vi "Calculate Zoom from ROI & Image Size.vi"(8 "Error In":errorcluster, 10 "ROI Descriptor":T1 {"Contours"."Type" items=["No Selection", "Point", "Line", "Rectangle", "Oval", "Polygon", "Freehand Region", "Annulus", "Unused2", "Unused3", "Broken Line", "Freehand Line", "Rotated Rectangle"]}, 11 "Displayed Image:Size":cluster{"Width":u32, "Height":u32}) -> (0 "Error Out":errorcluster, 2 "Center Position":cluster{dbl, dbl}, 3 "Zoom Factor":cluster{dbl, dbl})   [LabVIEW 2021, in "Image.lvlib"]
uses:
  <vilib>/Utility/error.llb/Error Cluster From Error Code.vi
  <vilib>/ErrorRing/Error Ring.xnode
  Image.lvlib
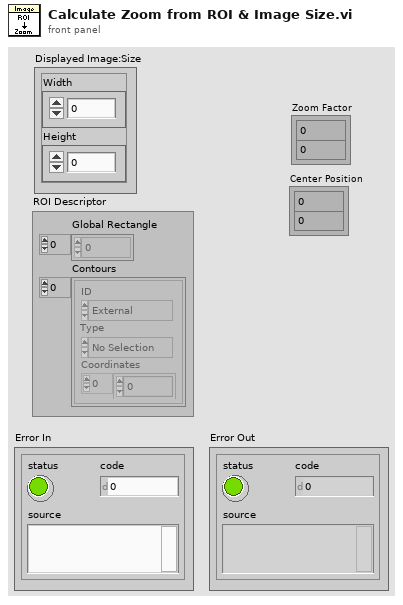
[diagram p1: front panel]
types:
  T1 = typedef "ROI Descriptor" = cluster{"Global Rectangle":i32[], "Contours":cluster{"ID":enum32{"External", "Internal"}, "Type":u32, "Coordinates":i32[]}[]}
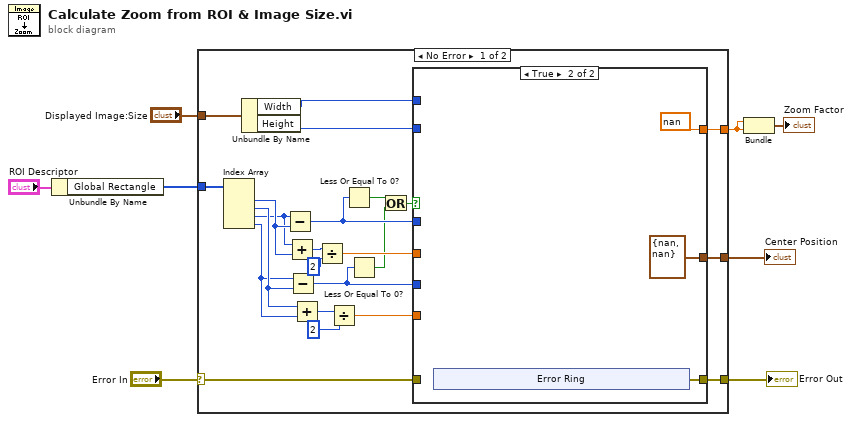
[diagram p0: block diagram]
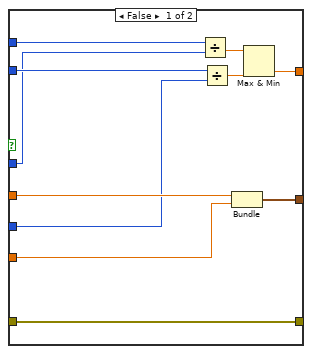
[diagram p2: hidden frame]
diagram:
  n1 = Unbundle By Name("ROI Descriptor") -> ("Global Rectangle"=w7:i32[])
  n2 = case shown="No Error" "Error In" {
    selector: "Error In" -> [w9 w50]
    tunnel: w7 -> [w31 _]
    tunnel: [w20 _] -> w6
    tunnel: [w19 _] -> w5
    tunnel: "Displayed Image:Size" -> [w18 _]
    tunnel: [w10 w50] -> w1
    frame No Error {
      n3 = Index Array(array=w31) -> (element #1=w26:i32, element #2=w30:i32, element #3=w25:i32, element #4=w29:i32)  [unwired: 4 in]
      n4 = Unbundle By Name(w18) -> ("Width"=w17:u32, "Height"=w16:u32)
      n5 = Subtract(x=w25, y=w26) -> (x-y=w15:i32)
      n6 = Add(x=w25, y=w26) -> (x+y=w24:i32)
      n7 = Subtract(x=w29, y=w30) -> (x-y=w14:i32)
      n8 = Add(x=w30, y=w29) -> (x+y=w28:i32)
      n9 = Divide(x=w24, y=2) -> (x/y=w22:dbl)
      n10 = Divide(x=w28, y=2) -> (x/y=w21:dbl)
      n11 = Less Or Equal To 0?(x=w15) -> (x <= 0?=w13:bool)
      n12 = Less Or Equal To 0?(x=w14) -> (x <= 0?=w12:bool)
      n13 = Or(x=w13, y=w12) -> (x .or. y?=w11:bool)
      n14 = case shown="True" w11 {
        tunnel: w22 -> [w40 _]
        tunnel: w21 -> [w39 _]
        tunnel: [w38 cluster{dbl, dbl} {nan, nan}] -> w20
        tunnel: [w37 nan] -> w19
        tunnel: w17 -> [w36 _]
        tunnel: w16 -> [w35 _]
        tunnel: w15 -> [w34 _]
        tunnel: w14 -> [w33 _]
        tunnel: [w32 w43] -> w10
        tunnel: w9 -> [w32 _]
        frame False {
          n15 = Divide(x=w36, y=w34) -> (x/y=w42:dbl)
          n16 = Divide(x=w35, y=w33) -> (x/y=w41:dbl)
          n17 = Bundle(w40, w39) -> (w38:cluster{dbl, dbl})  [unwired: 1 in]
          n18 = Max & Min(x=w42, y=w41) -> (min(x,y)=w37:dbl)  [unwired: 1 out]
        }
        frame True {
          n19 = xnode "Error Ring"() -> ("error out"=w43:errorcluster)
        }
      }
    }
    frame Error {
    }
  }
  "Center Position" <- w6
  "Error Out" <- w1
  n20 = Bundle(w5, w5) -> (→"Zoom Factor":cluster{dbl, dbl})  [unwired: 1 in]
